vi "Periodic Tasks.vi"(8 "error in":errorcluster) -> ()   [LabVIEW 2019]
doc: "This VI runs in parallel to other tasks. It can contain as many user-defined periodic loops as you need. These can carry out PID or other sorts of timed response."
uses:
  <vilib>/Rock Robotics/WPI/Utilities/WPI_GetSetVariantRefNum.vi
  <vilib>/Rock Robotics/Network Tables/NT Write Number.vi
  <vilib>/Rock Robotics/WPI/ThirdParty/Phoenix-LabVIEW/Motor Controller/Get/CTRE_Phoenix_MotorController_GetQuadratureData.vi
  <vilib>/Rock Robotics/Network Tables/NT Read Boolean.vi
  <vilib>/Rock Robotics/Network Tables/NT Read Number.vi
  <vilib>/addons/control/pid/NI_PID_pid.lvlib
  <vilib>/addons/control/pid/pid.llb/PID (DBL).vi
  Robot Global Data.vi
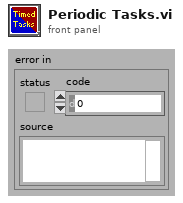
[diagram p1: front panel]
types:
  T1 = typedef "WPI_JoystickDevRef.ctl" = cluster{"Device":T2}
  T2 = typedef "WPI_JoystickDeviceEnum.ctl" = enum16{"USB 0", "USB 1", "USB 2", "USB 3", "USB 4", "USB 5"}
  T3 = typedef "WPI_MotorControlDeviceRef.ctl" = cluster{"DeviceStatus":errorcluster, "Type":T4, "PWM":cluster{"PWM Channel":T5, "DeadBand":T6}, "CAN":cluster{"Device Number":u8, "SetOutput VI Ref":variant, "GetOutput VI Ref":variant, "Enable VI Ref":variant, "Disable VI Ref":variant, "Data":variant}, "Invert":bool, "DIO PWM":cluster{"PWM \"Enable\" Channel":T5, "DIOChannel":T7, "PWM Rate":dbl}}
  T4 = typedef "WPI_MotorControlType.ctl" = enum16{"PWM", "CAN", "DIO PWM"}
  T5 = typedef "FPGA_DIOPWMChannel.ctl" = enum8{"PWM 0", "PWM 1", "PWM 2", "PWM 3", "PWM 4", "PWM 5", "PWM 6", "PWM 7", "PWM 8", "PWM 9", "PWM MXP 0", "PWM MXP 1", "PWM MXP 2", "PWM MXP 3", "PWM MXP 4", "PWM MXP 5", "PWM MXP 6", "PWM MXP 7", "PWM MXP 8", "PWM MXP 9", "Invalid"}
  T6 = typedef "WPI_PWMDeadband.ctl" = cluster{"Name":string, "maxPositivePwm":i32, "minPositivePwm":i32, "centerPwm":i32, "maxNegativePwm":i32, "minNegativePwm":i32, "angularRange":u16}
  T7 = typedef "FPGA_DIOChannel.ctl" = enum8{"DIO 0", "DIO 1", "DIO 2", "DIO 3", "DIO 4", "DIO 5", "DIO 6", "DIO 7", "DIO 8", "DIO 9", "DIO MXP 0", "DIO MXP 1", "DIO MXP 2", "DIO MXP 3", "DIO MXP 4", "DIO MXP 5", "DIO MXP 6", "DIO MXP 7", "DIO MXP 8", "DIO MXP 9", "DIO MXP 10", "DIO MXP 11", "DIO MXP 12", "DIO MXP 13", "DIO MXP 14", "DIO MXP 15", "SPI Port CS1", "SPI Port CS2", "SPI Port CS3", "SPI Port MISO", "SPI Port MOSI", "Invalid"}
  T8 = typedef "WPI_AnalogChannelDevRef.ctl" = cluster{"DevStatus":errorcluster, "Analog Channel":T9}
  T9 = typedef "FPGA_AIChannel.ctl" = enum8{"AI 0", "AI 1", "AI 2", "AI 3", "AI MXP 0", "AI MXP 1", "AI MXP 2", "AI MXP 3", "Invalid"}
  T10 = cluster{"Yaw":dbl, "Roll":dbl, "Pitch":dbl, "Heading":dbl, "Fused Heading":dbl}
  T11 = cluster{"proportional gain (Kc)":dbl, "integral time (Ti, min)":dbl, "derivative time (Td, min)":dbl}
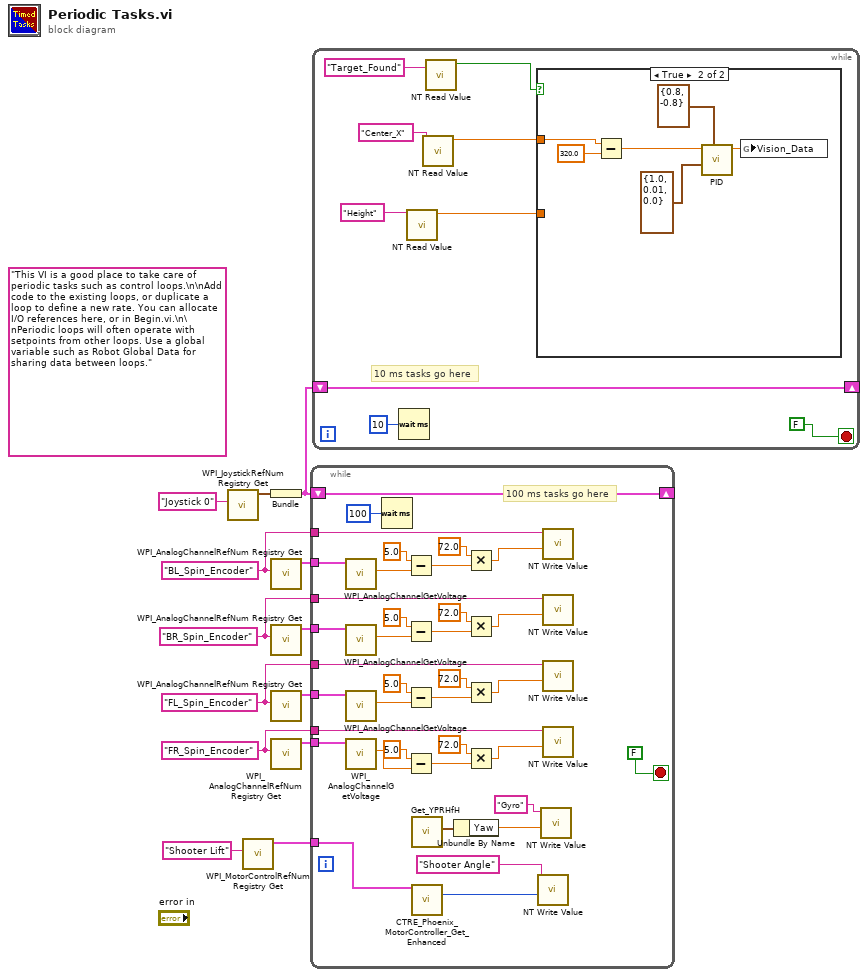
[diagram p0: block diagram]
diagram:
  w3 = "FL_Spin_Encoder" ("refnum name")
  w5 = "BL_Spin_Encoder" ("refnum name")
  w4 = "BR_Spin_Encoder" ("refnum name")
  w6 = "FR_Spin_Encoder" ("refnum name")
  (unwired) "This VI is a good place to take care of periodic tasks such as control loops.\n\nAdd code to the existing loops, or duplicate a loop to define a new rate. You can allocate I/O references here, or in Begin.vi.\n\nPeriodic loops will often operate with setpoints from other loops. Use a global variable such as Robot Global Data for sharing data between loops."
  n1 = call <vilib>:"WPI_JoystickRefNum Registry Get.vi"("refnum name"="Joystick 0") -> ("JoystickDevRef"=w12:T1)  [unwired: 1 in, 9 out]
  n2 = call <vilib>:"WPI_MotorControlRefNum Registry Get.vi"("refnum name"="Shooter Lift") -> ("MotorControlDevRef"=w1:T3)  [unwired: 9 in, 1 out]
  n3 = Bundle("JoystickDevRef"=w12) -> (w11:cluster{"JoystickDevRef":T1})  [unwired: 1 out]
  n4 = call <vilib>:"WPI_AnalogChannelRefNum Registry Get.vi"("refnum name"=w5) -> ("AIDeviceRef"=w7:T8)  [unwired: 9 in, 1 out]
  n5 = call <vilib>:"WPI_AnalogChannelRefNum Registry Get.vi"("refnum name"=w4) -> ("AIDeviceRef"=w8:T8)  [unwired: 9 in, 1 out]
  n6 = call <vilib>:"WPI_AnalogChannelRefNum Registry Get.vi"("refnum name"=w3) -> ("AIDeviceRef"=w9:T8)  [unwired: 9 in, 1 out]
  n7 = call <vilib>:"WPI_AnalogChannelRefNum Registry Get.vi"("refnum name"=w6) -> ("AIDeviceRef"=w10:T8)  [unwired: 9 in, 1 out]
  n8 = while {
    shift-right: [w48] -> _
    shift-left: w11 -> [w48]
    tunnel: w10 -> [w47]
    tunnel: w9 -> [w46]
    tunnel: w8 -> [w45]
    tunnel: w7 -> [w44]
    tunnel: w6 -> [w26]
    tunnel: w5 -> [w24]
    tunnel: w4 -> [w23]
    tunnel: w3 -> [w20]
    tunnel: w1 -> [w16]
    stop <- FALSE stop-if-true
    # "100 ms tasks go here"
    n9 = call <vilib>:"WPI_AnalogChannelGetVoltage.vi"("AIDeviceRef"=w44) -> ("Voltage"=w30:dbl)  [unwired: 8 in, 2 out]
    n10 = call <vilib>:"WPI_AnalogChannelGetVoltage.vi"("AIDeviceRef"=w45) -> ("Voltage"=w29:dbl)  [unwired: 8 in, 2 out]
    n11 = call <vilib>:"WPI_AnalogChannelGetVoltage.vi"("AIDeviceRef"=w46) -> ("Voltage"=w28:dbl)  [unwired: 8 in, 2 out]
    n12 = call <vilib>:"WPI_AnalogChannelGetVoltage.vi"("AIDeviceRef"=w47) -> ("Voltage"=w40:dbl)  [unwired: 8 in, 2 out]
    n13 = Wait (ms)(milliseconds to wait=u32 100) -> ()  [unwired: 1 out]
    n14 = Subtract(x=5.0, y=w30) -> (x-y=w31:dbl)
    n15 = Subtract(x=5.0, y=w29) -> (x-y=w36:dbl)
    n16 = Subtract(x=5.0, y=w28) -> (x-y=w37:dbl)
    n17 = Subtract(x=5.0, y=w40) -> (x-y=w43:dbl)
    n18 = call <vilib>:"Get_YPRHfH.vi"() -> ("YRPHfH"=w19:T10)  [unwired: 11 in]
    n19 = call-poly <vilib>:"CTRE_Phoenix_MotorController_Get_Enhanced.vi"("PhoenixMotorControlDevRef"=w16) -> ("Quadrature Position"=w15:i32)  [unwired: 11 in, 3 out]
    n20 = Unbundle By Name(w19) -> ("Yaw"=w18:dbl)
    n21 = Multiply(x=72.0 ("y"), y=w31) -> (x*y=w25:dbl)
    n22 = Multiply(x=72.0 ("y"), y=w36) -> (x*y=w22:dbl)
    n23 = Multiply(x=72.0 ("y"), y=w37) -> (x*y=w21:dbl)
    n24 = Multiply(x=72.0 ("y"), y=w43) -> (x*y=w27:dbl)
    n25 = call-poly <vilib>:"NT Write Value.vi"("Numeric"=w15, "Name"="Shooter Angle") -> ()  [unwired: 9 in, 1 out]
    n26 = call-poly <vilib>:"NT Write Value.vi"("Numeric"=w18, "Name"="Gyro") -> ()  [unwired: 9 in, 1 out]
    n27 = call-poly <vilib>:"NT Write Value.vi"("Numeric"=w25, "Name"=w24) -> ()  [unwired: 9 in, 1 out]
    n28 = call-poly <vilib>:"NT Write Value.vi"("Numeric"=w22, "Name"=w23) -> ()  [unwired: 9 in, 1 out]
    n29 = call-poly <vilib>:"NT Write Value.vi"("Numeric"=w21, "Name"=w20) -> ()  [unwired: 9 in, 1 out]
    n30 = call-poly <vilib>:"NT Write Value.vi"("Numeric"=w27, "Name"=w26) -> ()  [unwired: 9 in, 1 out]
  }
  n31 = while {
    shift-right: [w57] -> _
    shift-left: w11 -> [w57]
    stop <- FALSE stop-if-true
    # "10 ms tasks go here"
    n32 = Wait (ms)(milliseconds to wait=u32 10) -> ()  [unwired: 1 out]
    n33 = call-poly <vilib>:"NT Read Value.vi"("Name"="Height") -> ("Numeric"=w51:dbl)  [unwired: 9 in, 1 out]
    n34 = call-poly <vilib>:"NT Read Value.vi"("Name"="Center_X") -> ("Numeric"=w52:dbl)  [unwired: 9 in, 1 out]
    n35 = call-poly <vilib>:"NT Read Value.vi"("Name"="Target_Found") -> ("Boolean"=w53:bool)  [unwired: 9 in, 1 out]
    n36 = case shown="True" w53 {
      tunnel: w52 -> [_ w65]
      tunnel: w51 -> [_ _]
      frame False {
      }
      frame True {
        n37 = Subtract(x=w65, y=320.0) -> (x-y=w63:dbl)
        n38 = call-poly <vilib>:"PID.vi"("output range"=cluster{"output high":dbl, "output low":dbl} {"output high"=0.8, "output low"=-0.8}, "PID gains"=T11 {"proportional gain (Kc)"=1.0, "integral time (Ti, min)"=0.01, "derivative time (Td, min)"=0.0}, "setpoint"=w63) -> ("output"=w60:dbl)  [unwired: 7 in, 1 out]
        n39 = global write "Robot Global Data.vi" "Vision_Data"(w60) -> ()
      }
    }
  }
